vi "Start Undo.vi"(8 "error in (no error)":errorcluster, 10 "Name":string, 11 "CSM-Helper in":refnum<class "CSM-Helper.lvclass">) -> (0 "error out":errorcluster, 3 "CSM-Helper out":refnum<class "CSM-Helper.lvclass">)   [LabVIEW 2017, in "CSM-Helper.lvclass"]
doc: "### Start Undo.vi\n\n-- <b>Controls</b> --\n- <b>Name</b>:\n- <b>CSM-Helper in</b>: CSMHelper input\n\n-- <b>Indicators</b> --\n- <b>CSM-Helper out</b>: CSMHelper output"
uses:
  CSM-Helper.lvclass
  CSM-Helper.lvclass/CSM-Helper.ctl
  Properties/Read VI Ref.vi
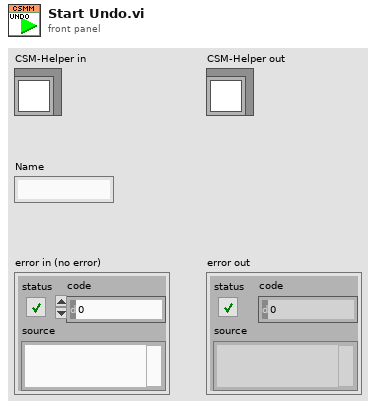
[diagram p1: front panel]
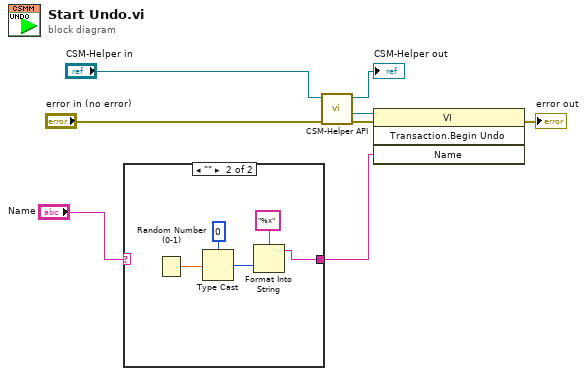
[diagram p0: block diagram]
diagram:
  n1 = case shown="\"\"" "Name" {
    selector: "Name" -> [w9 _]
    tunnel: [w9 w11] -> w2
    frame "False", Default {
    }
    frame "" {
      n2 = Random Number (0-1)() -> (number: 0 to 1=w14:dbl)
      n3 = Type Cast(type=u64 0 ("global-CSMQ FGV Change Flag"), x=w14) -> (*(type *) &x=w12:u64)
      n4 = Format Into String(format string="%x", w12) -> (resulting string=w11:string)  [unwired: 2 in, 1 out]
    }
  }
  n5 = call-poly "CSM-Helper API.vi"("error in (no error)"="error in (no error)", "CSM-Helper in"="CSM-Helper in") -> ("error out"=w7:errorcluster, "VI"=w1:refnum<vi>, "CSM-Helper out"=→"CSM-Helper out":refnum<class "CSM-Helper.lvclass">)  [unwired: 7 in]
  n6 = invoke class="VI" method="Transaction.Begin Undo"(reference=w1, error in=w7, "Name"=w2) -> (error out=→"error out":errorcluster)  [unwired: 1 in, 3 out]
